vi "WebView2Browser.vi"() -> ()   [LabVIEW 2020]
uses:
  D:/dev/WinFormsApp/WinFormsControls/bin/Release/WinFormsControls.dll
panel:
  in  "WebView2Control":refnum<k24>(container)
  out "Is browser initialized?":bool
  in  "Navigate":bool
  in  "url":string="https://www.ni.com/labview"
  in  "stop":bool
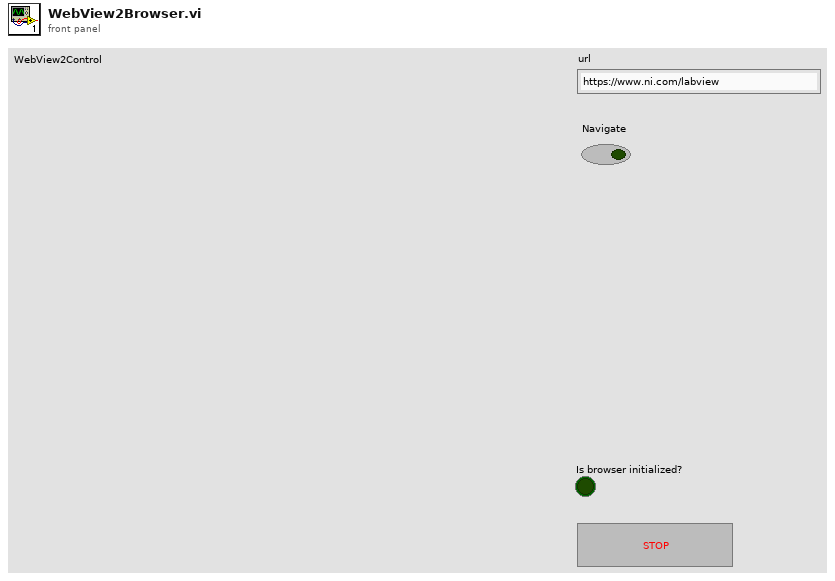
[diagram p1: front panel]
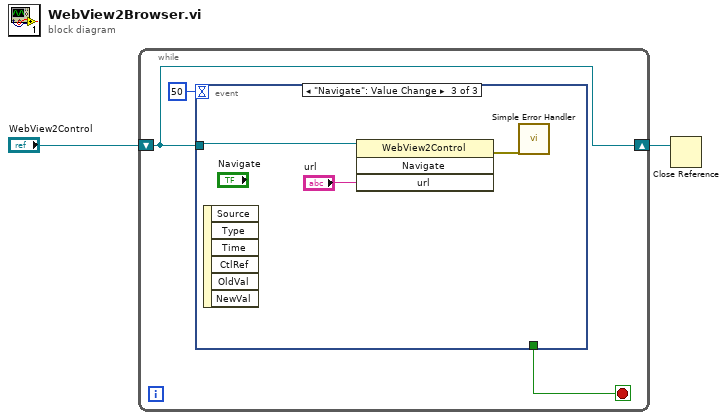
[diagram p0: block diagram]
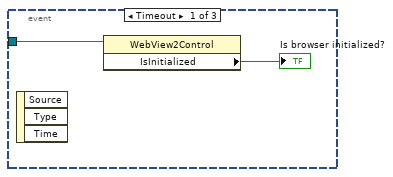
[diagram p2: hidden frame]
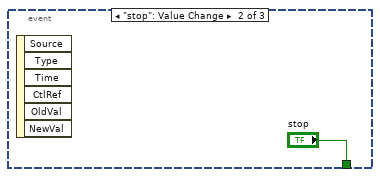
[diagram p3: hidden frame]
diagram:
  n1 = while {
    shift-right: [w4] -> w2
    shift-left: "WebView2Control" -> [w4]
    stop <- w3 stop-if-true
    n2 = event shown="[2] \"Navigate\": Value Change" {
      selector: _ -> [_ _ _]
      dyn-events: _ -> [_ _ _]
      timeout: 50 -> [_ _ _]
      tunnel: [_ "stop" _] -> w3
      tunnel: w4 -> [w7 _ w11]
      event Timeout {
        n3 = event-data() -> ()  [unwired: 1 in, 3 out]
        n4 = property class="WebView2Control"(reference=w7) -> ("IsInitialized"=→"Is browser initialized?":bool)  [unwired: 1 in, 2 out]
      }
      event "stop": Value Change {
        n5 = event-data() -> ()  [unwired: 1 in, 6 out]
      }
      event "Navigate": Value Change {
        n6 = event-data() -> ()  [unwired: 1 in, 6 out]
        n7 = invoke class="WebView2Control" method="Navigate"(reference=w11, "url"="url") -> (error out=w9:errorcluster)  [unwired: 2 in, 3 out]
        n8 = call <vilib>:"Simple Error Handler.vi"("error in (no error)"=w9) -> ()  [unwired: 4 in, 5 out]
      }
    }
  }
  n9 = Close Reference(reference=w2) -> ()  [unwired: 1 in, 1 out]
